vi "xVDT Page.vi"(8 "error in (no error)":errorcluster, 11 "Node Ptr":T1 format="%.0x") -> (0 "error out":errorcluster)   [LabVIEW 2011, in "Sensor Simulation Custom Device.lvlib"]
uses:
  Sensor Simulation Custom Device.lvlib
  <vilib>/NI Veristand/Custom Device API/Custom Device Item Ref.ctl
  Real-Time/TypeDefs/SensorType.ctl
  Global.vi
  <vilib>/NI Veristand/Custom Device API/Get Item Property (Variant).vi
  <vilib>/NI Veristand/Custom Device API/Get Item Property (Double).vi
  <vilib>/NI Veristand/Custom Device API/Set Item Property (Double).vi
  <vilib>/NI Veristand/Custom Device API/Custom Device API.lvlib
panel:
  in  "SHDocVw.IWebBrowser2":refnum<k7>(container)
  in  "Units":string caption="Position Units"
  in  "TransRatio":dbl caption="Transfer Ratio (V/V)"
  in  "Sens":dbl caption="Differential Sensitivity (V/V/units)"
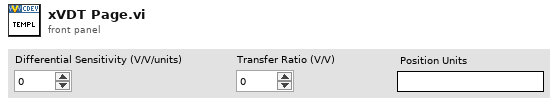
[diagram p1: front panel]
types:
  T1 = typedef "Custom Device API.lvlib/Custom Device Item Ref.ctl" = u64
  T2 = typedef "Sensor Simulation Custom Device.lvlib/SensorType.ctl" = enum16{"Resolver", "4 Wire xVDT", "5 Wire xVDT", "Invalid"}
  T3 = typedef "Custom Device API.lvlib/Custom Device Channel.ctl" = cluster{"Type":T4, "Units":string, "Default Value":dbl, "Faultable":bool, "Scalable":bool}
  T4 = typedef "Custom Device API.lvlib/Custom Device Channel Type.ctl" = enum16{"Input", "Output"}
  T5 = typedef "Custom Device API.lvlib/Custom Device Commands.ctl" = enum16{"Default", "Item renamed", "Shutdown", "Dynamic button pressed"}
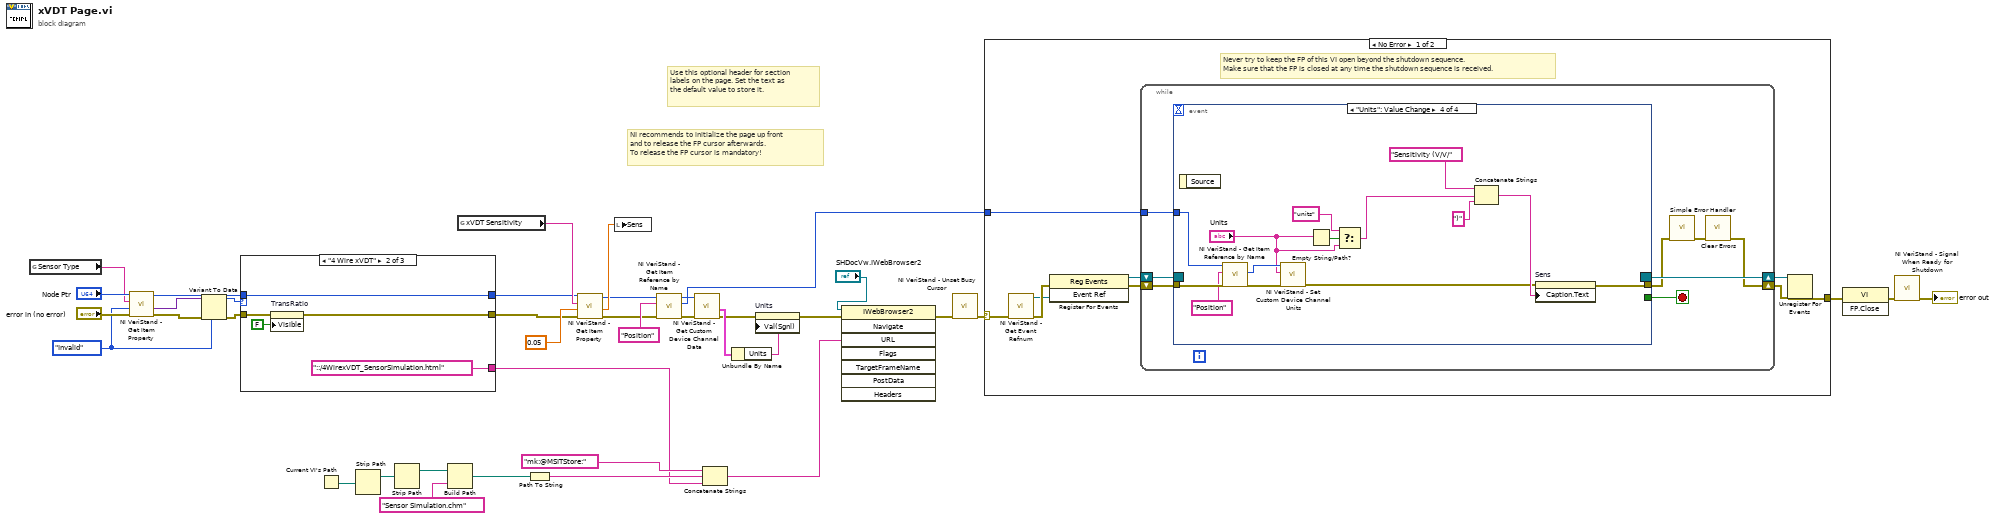
[diagram p0: block diagram]
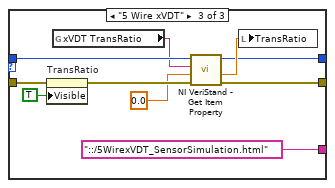
[diagram p3: hidden frame]
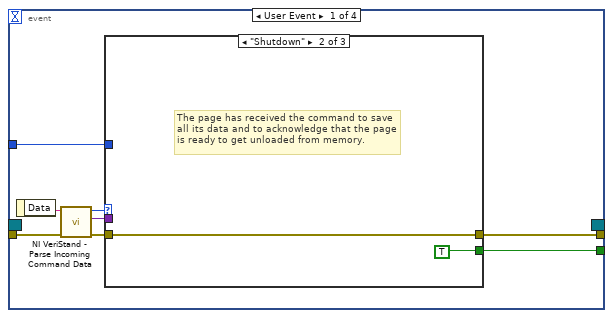
[diagram p4: hidden frame]
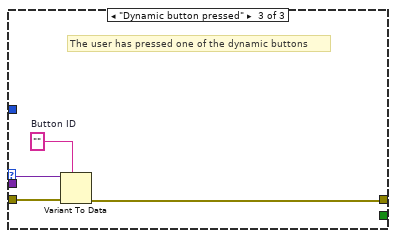
[diagram p6: hidden frame]
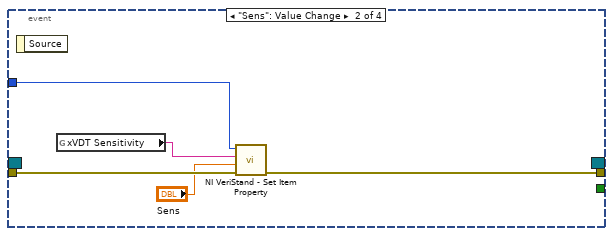
[diagram p7: hidden frame]
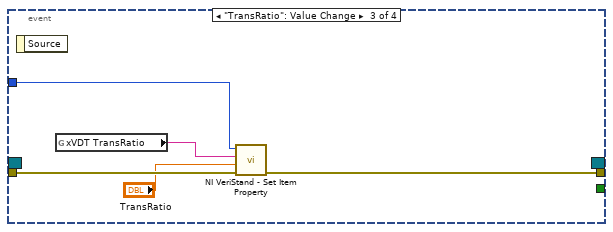
[diagram p8: hidden frame]
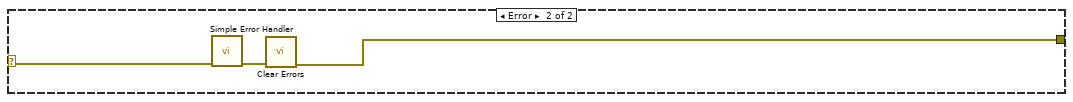
[diagram p9: hidden frame]
diagram:
  w3 = SensorType."Invalid" ("Sensor")
  # "Use this optional header for section labels on the page. Set the text as the default value to store it."
  # "NI recommends to initialize the page up front\nand to release the FP cursor afterwards.\nTo release the FP cursor is mandatory!"
  n1 = global read "Global.vi" "Sensor Type"() -> (w31:string)
  n2 = call-poly <vilib>:"NI VeriStand - Get Item Property.vi"("error in (no error)"="error in (no error)", "Default Value"=w3, "Property Name"=w31, "Item Ref in"="Node Ptr") -> ("error out"=w6:errorcluster, "Value"=w4:variant, "Item Ref out"=w30:T1)  [unwired: 4 in, 1 out]
  n3 = Variant To Data(error in=w6, type=w3, Variant=w4) -> (data=w2:T2, error out=w5:errorcluster)
  n4 = case shown="\"4 Wire xVDT\"" w2 {
    tunnel: w30 -> [w40 w43 w54]
    tunnel: [w40 w43 w51] -> w29
    tunnel: [w41 w44 w50] -> w28
    tunnel: w5 -> [w41 w46 w49]
    tunnel: [_ "::/4WirexVDT_SensorSimulation.html" ("name or relative path") "::/5WirexVDT_SensorSimulation.html" ("name or relative path")] -> w1
    frame Default {
    }
    frame "4 Wire xVDT" {
      n5 = property on="TransRatio" class="DigNum (strict)"(error in=w46, "Visible"=FALSE) -> (error out=w44:errorcluster)  [unwired: 1 in, 1 out]
    }
    frame "5 Wire xVDT" {
      n6 = property on="TransRatio" class="DigNum (strict)"(error in=w49, "Visible"=TRUE) -> (error out=w56:errorcluster)  [unwired: 1 in, 1 out]
      n7 = global read "Global.vi" "xVDT TransRatio"() -> (w53:string)
      n8 = call-poly <vilib>:"NI VeriStand - Get Item Property.vi"("error in (no error)"=w56, "Default Value"=0.0, "Property Name"=w53, "Item Ref in"=w54) -> ("error out"=w50:errorcluster, "Value"=w52:dbl, "Item Ref out"=w51:T1)  [unwired: 4 in, 1 out]
      n9 = local write "TransRatio"(w52) -> ()
    }
  }
  n10 = Current VI's Path() -> (path=w18:path)
  n11 = Strip Path(path=w18) -> (stripped path=w17:path)  [unwired: 1 out]
  n12 = Strip Path(path=w17) -> (stripped path=w12:path)  [unwired: 1 out]
  n13 = Build Path(base path=w12, name or relative path="Sensor Simulation.chm") -> (appended path=w14:path)
  n14 = global read "Global.vi" "xVDT Sensitivity"() -> (w34:string)
  n15 = Path To String(path=w14) -> (string=w15:string)
  n16 = call-poly <vilib>:"NI VeriStand - Get Item Property.vi"("error in (no error)"=w28, "Default Value"=0.05, "Property Name"=w34, "Item Ref in"=w29) -> ("error out"=w20:errorcluster, "Value"=w33:dbl, "Item Ref out"=w19:T1)  [unwired: 4 in, 1 out]
  n17 = local write "Sens"(w33) -> ()
  n18 = call <vilib>:"NI VeriStand - Get Item Reference by Name.vi"("error in (no error)"=w20, "Item Name"="Position", "Parent Ref in"=w19) -> ("error out"=w26:errorcluster, "Item Ref"=w25:T1, "Parent Ref out"=w24:T1)  [unwired: 5 in, 1 out]
  n19 = call <vilib>:"NI VeriStand - Get Custom Device Channel Data.vi"("error in (no error)"=w26, "Channel Ref in"=w25) -> ("error out"=w22:errorcluster, "Channel"=w23:T3)  [unwired: 4 in, 4 out]
  n20 = Concatenate Strings("mk:@MSITStore:" ("string"), w15, w1) -> (w8:string)
  n21 = Unbundle By Name(w23) -> ("Units"=w21:string)
  n22 = property on="Units" class="Str"(error in=w22, "Val(Sgnl)"=w21) -> (error out=w9:errorcluster)  [unwired: 1 in, 1 out]
  n23 = invoke class="IWebBrowser2" method="Navigate"(reference="SHDocVw.IWebBrowser2", error in=w9, "URL"=w8) -> (error out=w10:errorcluster)  [unwired: 5 in, 7 out]
  n24 = call <vilib>:"NI VeriStand - Unset Busy Cursor.vi"("error in (no error)"=w10) -> ("error out"=w36:errorcluster)  [unwired: 10 out]
  n25 = case shown="No Error" w36 {
    selector: w36 -> [w57 w115]
    tunnel: [w62 w113] -> w39
    tunnel: w24 -> [w58 _]
    frame No Error {
      # "Never try to keep the FP of this VI open beyond the shutdown sequence.\nMake sure that the FP is closed at any time the shutdown sequence is received."
      n26 = call <vilib>:"NI VeriStand - Get Event Refnum.vi"("error in (no error)"=w57) -> ("error out"=w65:errorcluster, "Event Ref"=w61:refnum<user-event>)  [unwired: 9 out]
      n27 = register-events(error in=w65, w61) -> (reference out=w59:refnum<event-registration>, error out=w60:errorcluster)  [unwired: 1 in]
      n28 = while {
        tunnel: w58 -> [w69]
        shift-right: [w66] -> w63
        shift-left: w60 -> [w72]
        shift-right: [w73] -> w64
        shift-left: w59 -> [w71]
        stop <- w70 stop-if-true
        n29 = event shown="[3] \"Units\": Value Change" {
          selector: w71 -> [_ _ _ _]
          dyn-events: [_ _ _ _] -> w73
          timeout: _ -> [_ _ _ _]
          tunnel: w72 -> [w81 w93 w98 w112]
          tunnel: [w77 _ _ _] -> w70
          tunnel: [w76 w90 w96 w104] -> w68
          tunnel: w69 -> [w75 w92 w97 w111]
          event User Event {
            n30 = event-data() -> ("Data"=w80:string)  [unwired: 1 out]
            n31 = call <vilib>:"NI VeriStand - Parse Incoming Command Data.vi"("error in (no error)"=w81, "Incoming data"=w80) -> ("error out"=w79:errorcluster, "Outgoing data"=w74:variant, "Action"=w78:T5)  [unwired: 7 out]
            n32 = case shown="\"Shutdown\"" w78 {
              tunnel: w79 -> [w82 w83 w88]
              tunnel: [_ TRUE _] -> w77
              tunnel: [w82 w83 w85] -> w76
              tunnel: w75 -> [_ _ _]
              tunnel: w74 -> [_ _ w87]
              frame "Default", Default {
              }
              frame "Shutdown" {
                # "The page has received the command to save all its data and to acknowledge that the page is ready to get unloaded from memory."
              }
              frame "Dynamic button pressed" {
                w86 = ""  # Button ID
                # "The user has pressed one of the dynamic buttons"
                n33 = Variant To Data(error in=w88, type=w86, Variant=w87) -> (error out=w85:errorcluster)  [unwired: 1 out]
              }
            }
          }
          event "Sens": Value Change {
            n34 = event-data() -> ()  [unwired: 2 out]
            n35 = global read "Global.vi" "xVDT Sensitivity"() -> (w89:string)
            n36 = call-poly <vilib>:"NI VeriStand - Set Item Property.vi"("error in (no error)"=w93, "Value"="Sens", "Property Name"=w89, "Item Ref in"=w92) -> ("error out"=w90:errorcluster)  [unwired: 5 in, 2 out]
          }
          event "TransRatio": Value Change {
            n37 = event-data() -> ()  [unwired: 2 out]
            n38 = global read "Global.vi" "xVDT TransRatio"() -> (w95:string)
            n39 = call-poly <vilib>:"NI VeriStand - Set Item Property.vi"("error in (no error)"=w98, "Value"="TransRatio", "Property Name"=w95, "Item Ref in"=w97) -> ("error out"=w96:errorcluster)  [unwired: 5 in, 2 out]
          }
          event "Units": Value Change {
            n40 = event-data() -> ()  [unwired: 2 out]
            n41 = call <vilib>:"NI VeriStand - Get Item Reference by Name.vi"("error in (no error)"=w112, "Item Name"="Position", "Parent Ref in"=w111) -> ("error out"=w109:errorcluster, "Item Ref"=w108:T1)  [unwired: 5 in, 2 out]
            n42 = call <vilib>:"NI VeriStand - Set Custom Device Channel Units.vi"("error in (no error)"=w109, "Units"="Units", "Channel Ref in"=w108) -> ("error out"=w99:errorcluster)  [unwired: 7 in, 1 out]
            n43 = Empty String/Path?(string/path="Units") -> (empty?=w107:bool)
            n44 = Select(t="units" ("Item Name"), s=w107, f="Units") -> (s? t:f=w100:string)
            n45 = Concatenate Strings("Sensitivity (V/V/" ("string"), w100, ")" ("string")) -> (w101:string)
            n46 = property on="Sens" class="DigNum (strict)"(error in=w99, "Caption.Text"=w101) -> (error out=w104:errorcluster)  [unwired: 1 in, 1 out]
          }
        }
        n47 = call <vilib>:"Simple Error Handler.vi"("error in (no error)"=w68) -> ("error out"=w67:errorcluster)  [unwired: 1 in, 7 out]
        n48 = call <vilib>:"Clear Errors.vi"("error in (no error)"=w67) -> ("error out"=w66:errorcluster)  [unwired: 6 out]
      }
      n49 = Unregister For Events(event registration refnum=w64, error in=w63) -> (error out=w62:errorcluster)
    }
    frame Error {
      n50 = call <vilib>:"Simple Error Handler.vi"("error in (no error)"=w115) -> ("error out"=w114:errorcluster)  [unwired: 1 in, 7 out]
      n51 = call <vilib>:"Clear Errors.vi"("error in (no error)"=w114) -> ("error out"=w113:errorcluster)  [unwired: 6 out]
    }
  }
  n52 = invoke class="VI" method="FP.Close"(error in=w39) -> (error out=w38:errorcluster)  [unwired: 2 in, 2 out]
  n53 = call <vilib>:"NI VeriStand - Signal When Ready for Shutdown.vi"("error in (no error)"=w38) -> ("error out"=→"error out":errorcluster)  [unwired: 10 out]
